vi "ConvertToVoltPolymorphic.vi"   [LabVIEW 2016]
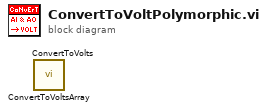
[diagram p0: block diagram]
diagram:
  n1 = call "ConvertToVoltsArray.vi"() -> ()  [unwired: 11 in, 1 out]
  n2 = call "ConvertToVolts.vi"() -> ()  [unwired: 11 in, 1 out]
